vi "HMI VI.vi"() -> ()   [LabVIEW 2014]
panel:
  in  "Reboot":bool
  in  "정지":bool
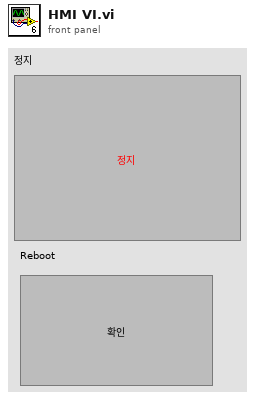
[diagram p1: front panel]
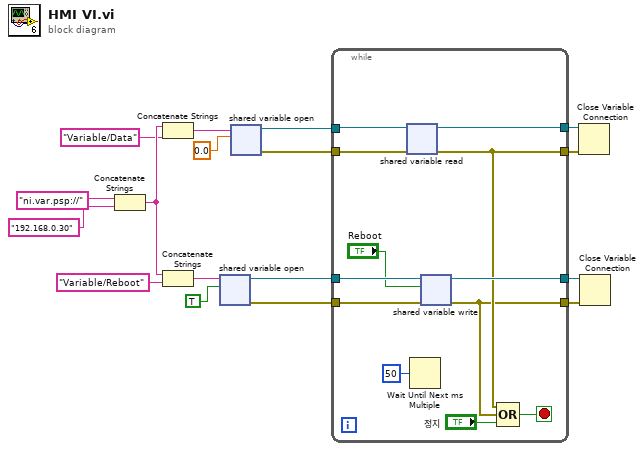
[diagram p0: block diagram]
diagram:
  n1 = Concatenate Strings("ni.var.psp://", "192.168.0.30" ("문자열")) -> (w12:string)
  n2 = Concatenate Strings(w12, "Variable/Data") -> (w13:string)
  n3 = Concatenate Strings(w12, "Variable/Reboot") -> (w15:string)
  n4 = shared-variable-open(w15, TRUE) -> (w7:refnum<k21>, w5:errorcluster)  [unwired: 2 in]
  n5 = shared-variable-open(w13, 0.0) -> (w8:refnum<k21>, w6:errorcluster)  [unwired: 2 in]
  n6 = while {
    tunnel: w8 -> [w29]
    tunnel: w7 -> [w27]
    tunnel: w6 -> [w28]
    tunnel: w5 -> [w26]
    tunnel: [w24] -> w3
    tunnel: [w22] -> w4
    tunnel: [w23] -> w1
    tunnel: [w21] -> w2
    stop <- w19 stop-if-true
    n7 = shared-variable-read(w29, w28) -> (w24:refnum<k21>, w22:errorcluster)  [unwired: 2 out]
    n8 = Wait Until Next ms Multiple(millisecond multiple=u32 50 ("ms 배수")) -> ()  [unwired: 1 out]
    n9 = shared-variable-write(w27, w26, "Reboot") -> (w23:refnum<k21>, w21:errorcluster)
    n10 = Compound Arithmetic op=OR(w22, w21, "정지") -> (w19:bool)
  }
  n11 = Close Variable Connection(8:w4, 11:w3) -> ()  [unwired: 1 out]
  n12 = Close Variable Connection(8:w2, 11:w1) -> ()  [unwired: 1 out]
